vi "Set Configuration.vi"(8 "error in (no error)":errorcluster, 11 "Digital PWM Input in":refnum<class "Digital PWM Input.lvclass">) -> (0 "error out":errorcluster, 3 "Digital PWM Input out":refnum<class "Digital PWM Input.lvclass">)   [LabVIEW 2015, in "Digital PWM Input.lvclass"]
uses:
  Digital PWM Input.lvclass
  IO Class/Type.ctl
  FPGA Addon Input/FPGA Addon Input.lvclass
  IO Class/IO Class.lvclass
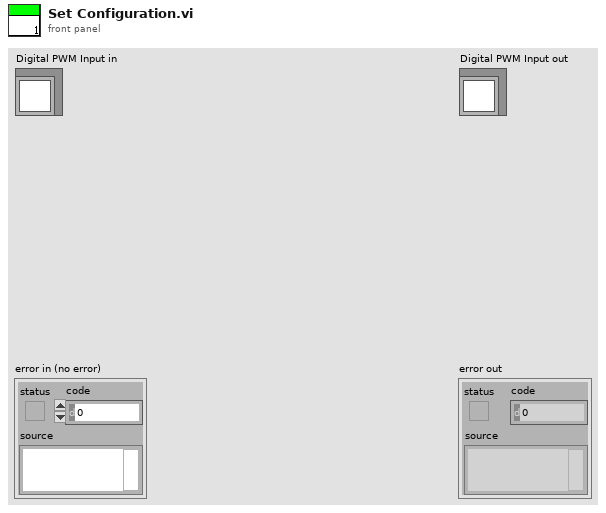
[diagram p1: front panel]
types:
  T1 = typedef "IO Class.lvclass/Type.ctl" = cluster{"Type":string}
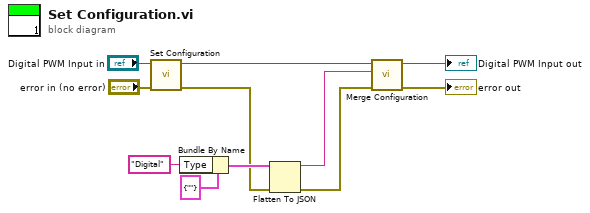
[diagram p0: block diagram]
diagram:
  n1 = call-parent "Set Configuration.vi"("error in (no error)"="error in (no error)", "FPGA Addon Input in"="Digital PWM Input in") -> ("error out"=w5:errorcluster, "FPGA Addon Input out"=w7:refnum<class "Digital PWM Input.lvclass">)  [unwired: 8 in]
  n2 = Bundle By Name(cluster=T1 {"Type"=""} ("Type"), "Type"="Digital") -> (w8:T1)
  n3 = Flatten To JSON(anything=w8, error in (no error)=w5) -> (JSON string=w6:string, 11:w4:errorcluster)  [unwired: 1 in]
  n4 = call "Merge Configuration.vi"("error in (no error)"=w4, "Additional Configuration"=w6, "IO Class in"=w7) -> ("error out"=→"error out":errorcluster, "IO Class out"=→"Digital PWM Input out":refnum<class "Digital PWM Input.lvclass">)  [unwired: 7 in]
